vi "PH_Sequencer_Watch.PC PPInternalTiming.vi"(0 "i ref in":refnum<vi>, 3 "Remaining Time [s]":dbl=30.0, 4 "no link?":bool, 5 "error in (no error)":errorcluster) -> (14 "i ref out":refnum<vi>, 19 "error out":errorcluster)   [LabVIEW 2014, in "PH_Sequencer_Watch.lvlib"]
doc: "This VI writes the remaining waiting time of the PU to own attributes and the GUI elements."
uses:
  PH_Sequencer_Watch.lvlib
  PH_Common/PH_Common.lvlib
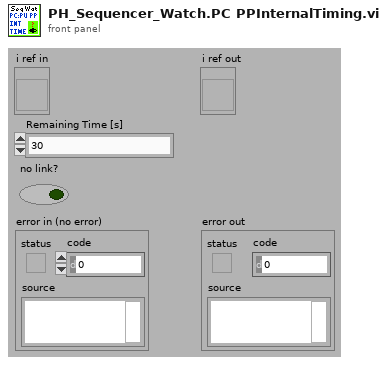
[diagram p1: front panel]
types:
  T1 = typedef "PH_Sequencer_Watch.lvlib/PH_Sequencer_Watch.i attribute.ctl" = cluster{"GUI Refs":cluster{"Shot ID":refnum<vi>, "Sequencer SM State":refnum<vi>, "Remaining Time":refnum<vi>, "PHELIX_Timing_T2":refnum<vi>, "T2-Unit-Dummy":refnum<vi>, "fs_Synchrolock_Watch":refnum<vi>, "Experiment_Vacuum_Control_Experiment":refnum<vi>}, "Status Synchrolock":T2, "Exp - Pressure":dbl, "Exp - Limit":dbl, "Heads":T3[], "Refs BooleanState":refnum<vi>[]}
  T2 = typedef "PH_StatusHandler.lvlib/PH_StatusHandler.Status.ctl" = i16
  T3 = typedef "PH_Sequencer_Watch.lvlib/PH_Sequencer_Watch.Head Information.ctl" = cluster{"Ref Volt":refnum<vi>, "PU":T4}
  T4 = typedef "PH_PP_Common.lvlib/PH_PP_Common.PUs.ctl" = enum16{"no Info", "PA-19mm-1", "PA-19mm-2", "PA-45mm-PILC", "PA-45mm-MAIN", "MA-PU-1", "MA-PU-2", "MA-PU-3", "MA-PU-4", "MA-PU-5", "MA-PU-6", "MA-FR", "MA-PILC", "PA-45mm-DP"}
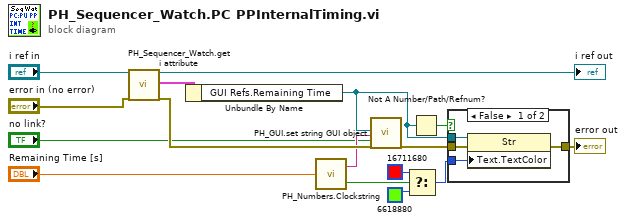
[diagram p0: block diagram]
diagram:
  n1 = call "PH_Sequencer_Watch.get i attribute.vi"("i ref in"="i ref in", "error in (no error)"="error in (no error)") -> ("i ref out"=→"i ref out":refnum<vi>, "i attribute"=w16:T1, "error out"=w12:errorcluster)  [unwired: 15 in]
  n2 = Unbundle By Name(w16) -> ("GUI Refs.Remaining Time"=w5:refnum<vi>)
  n3 = call "PH_Numbers.Clockstring.vi"("Time [s]"="Remaining Time [s]") -> ("Clock String"=w9:string, "<0?"=w3:bool)
  n4 = call "PH_GUI.set string GUI object.vi"("GUI object Ref"=w5, "Text"=w9, "Blinking? (false)"="no link?", "error in"=w12) -> ("error out"=w11:errorcluster)  [unwired: 15 in]
  n5 = Select(t=u32 16711680 ("Color Box"), s=w3, f=u32 6618880 ("Color Box")) -> (s? t:f=w2:u32)
  n6 = Not A Number/Path/Refnum?(number/path/refnum=w5) -> (NaN/Path/Refnum?=w6:bool)
  n7 = case shown="False" w6 {
    tunnel: w11 -> [w20 w21]
    tunnel: [w19 w21] -> w7
    tunnel: w5 -> [w18 _]
    tunnel: w2 -> [w17 _]
    frame False {
      n8 = property class="Str"(reference=w18, error in=w20, "Text.TextColor"=w17) -> (error out=w19:errorcluster)  [unwired: 1 out]
    }
    frame True {
    }
  }
  "error out" <- w7
